vi "Output.vi"(8 "error in (no error)":errorcluster, 10 "SignalGeneratorParameter":cluster{"Frequency":dbl, "Amplitude":dbl}={"Frequency"=10.0, "Amplitude"=1.0}, 11 "Generator in":refnum<class "Generator.lvclass">) -> (0 "error out":errorcluster, 2 "Waveform":waveform(dbl), 3 "Generator out":refnum<class "Generator.lvclass">)   [LabVIEW 2013, in "Generator.lvclass"]
uses:
  Generator.lvclass
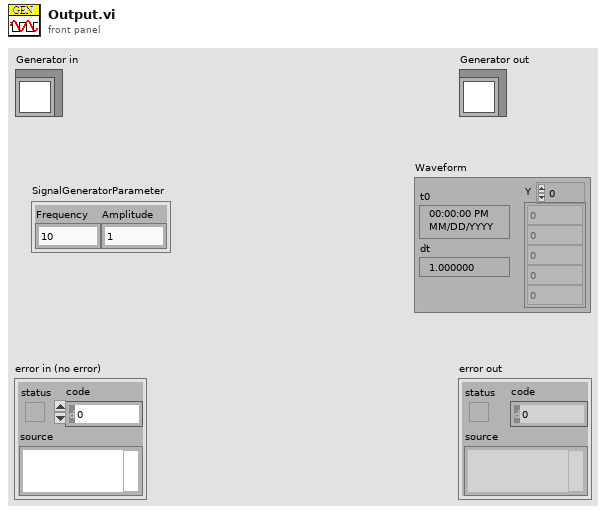
[diagram p1: front panel]
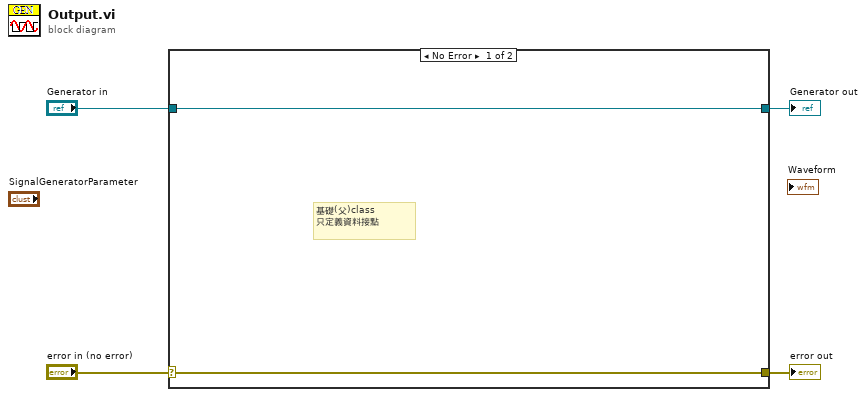
[diagram p0: block diagram]
diagram:
  n1 = case shown="No Error" "error in (no error)" {
    selector: "error in (no error)" -> [w5 w8]
    tunnel: [w5 w8] -> w3
    tunnel: [w6 w7] -> w1
    tunnel: "Generator in" -> [w6 w7]
    frame No Error {
      # "基礎(父)class\n只定義資料接點"
    }
    frame Error {
    }
  }
  "error out" <- w3
  "Generator out" <- w1
